vi "ConsoleRedErrors.vi"(8 "Text.Selection:End":u32, 9 "Front Panel":refnum<vi>, 10 "Console in":string, 11 "String in":refnum<vi>) -> (2 "Array":T1(array[cluster]), 3 "Console":string)   [LabVIEW 2021]
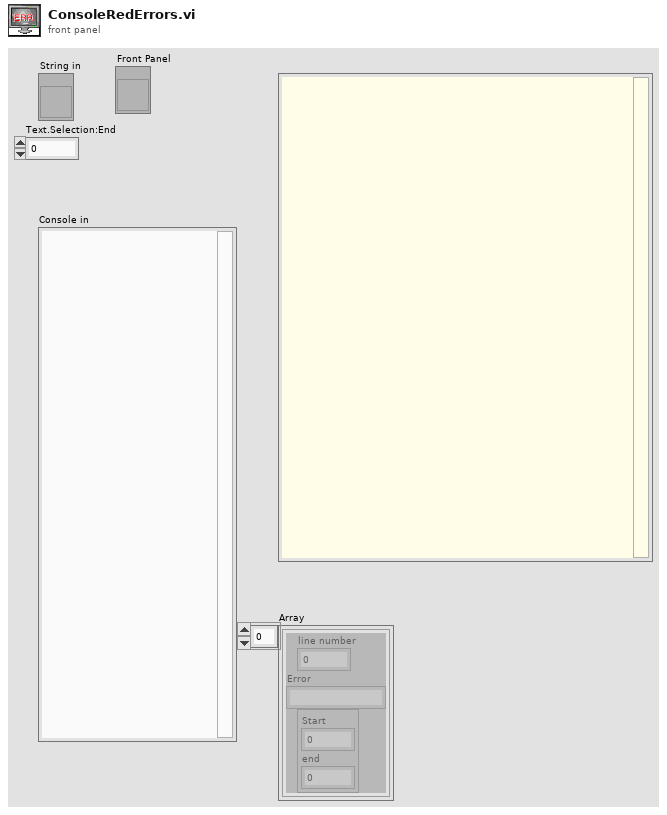
[diagram p1: front panel]
types:
  T1 = cluster{"line number":i32, "Error":string, cluster{"Start":i32, "end":i32}}[]
  T2 = cluster{i32, "Console in":string, cluster{i32, "offset past match":i32}}
  T3 = cluster{"line number":i32, "Error":string, cluster{"Start":i32, "end":i32}}
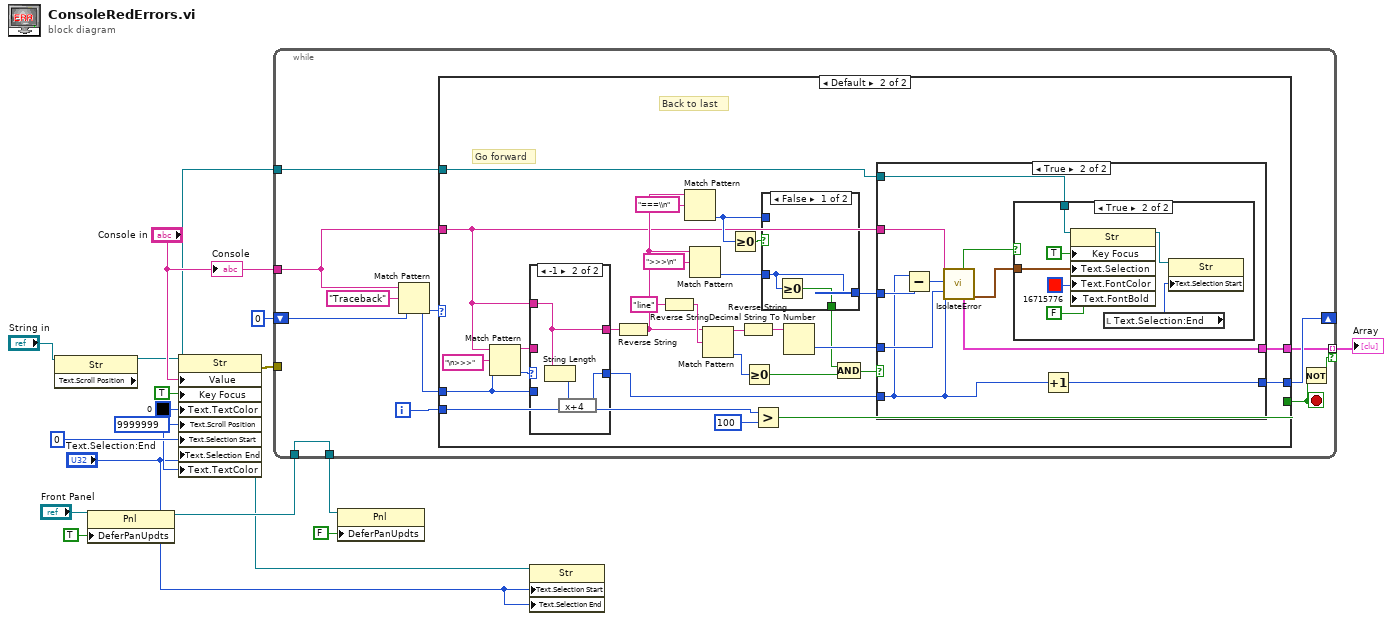
[diagram p0: block diagram]
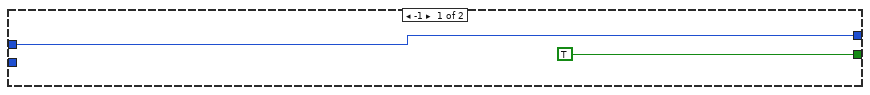
[diagram p2: hidden frame]
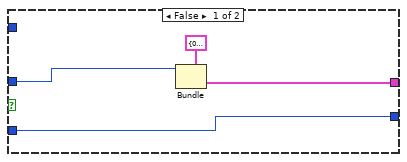
[diagram p3: hidden frame]
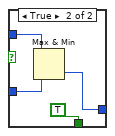
[diagram p6: hidden frame]
diagram:
  w3 = u32 0 ("Text.Text Colors:Text Color")
  n1 = property on="Property Node" class="Str" props=["Text", "Scroll Position"](reference="String in") -> (reference out=w10:refnum<vi>)  [unwired: 1 in, 2 out]
  n2 = property class="Pnl"(reference="Front Panel", "DeferPanUpdts"=TRUE ("Defer Panel Updates")) -> (reference out=w5:refnum<vi>)  [unwired: 1 in, 1 out]
  n3 = property on="Property Node" class="Str"(reference=w10, "Value"="Console in", "Key Focus"=TRUE, "Text.TextColor"=w3, "Text.Scroll Position"=u32 9999999, "Text.Selection Start"=u32 0 ("Text.Selection:Start"), "Text.Selection End"="Text.Selection:End", "Text.TextColor"=w3) -> (reference out=w2:refnum<vi>, error out=w14:errorcluster)  [unwired: 1 in]
  n4 = while {
    tunnel: "Console in" -> [w27]
    shift-right: [w25] -> _
    shift-left: 0 ("offset past match") -> [w26]
    tunnel: [w23] -> w16 mode=indexing if=w21
    tunnel: w14 -> [_]
    tunnel: w10 -> [w19]
    tunnel: [w18] -> w6
    tunnel: w5 -> [w18]
    i -> [w20]
    stop <- w22 stop-if-true
    n5 = Match Pattern(string=w27, regular expression="Traceback", offset (0)=w26) -> (offset past match=w24:i32)  [unwired: 3 out]
    n6 = case shown="Default" w24 {
      tunnel: w24 -> [w29 w32]
      tunnel: w27 -> [_ w35]
      tunnel: [w29 w46] -> w25
      tunnel: [TRUE w43] -> w22
      tunnel: [_ w52] -> w23
      tunnel: w20 -> [_ w44]
      tunnel: w19 -> [_ w31]
      frame -1 {
      }
      frame Default {
        # "Back to last"
        # "Go forward"
        n7 = Match Pattern(string=w35, regular expression="\n>>>", offset (0)=w32) -> (before substring=w33:string, offset past match=w37:i32)  [unwired: 2 out]
        n8 = case shown="-1" w37 {
          selector: w37 -> [w81 _]
          tunnel: [w82 w85] -> w36
          tunnel: w35 -> [_ w85]
          tunnel: [w81 w83] -> w34
          tunnel: w33 -> [w82 _]
          tunnel: w32 -> [_ _]
          frame Default {
          }
          frame -1 {
            n9 = String Length(string=w85) -> (length=w84:i32)
            n10 = expression code="x+4"(w84) -> (w83:i32)
          }
        }
        n11 = Reverse String(1:w36) -> (0:w50:string)
        n12 = Reverse String(1:"line" ("regular expression")) -> (0:w57:string)
        n13 = Match Pattern(string=w50, regular expression="===\\n") -> (offset past match=w49:i32)  [unwired: 1 in, 3 out]
        n14 = Match Pattern(string=w50, regular expression=">>>\n") -> (offset past match=w39:i32)  [unwired: 1 in, 3 out]
        n15 = Match Pattern(string=w50, regular expression=w57) -> (before substring=w56:string, offset past match=w42:i32)  [unwired: 1 in, 2 out]
        n16 = Greater Or Equal To 0?(x=w49) -> (x >= 0?=w48:bool)
        n17 = Reverse String(1:w56) -> (0:w55:string)
        n18 = Greater Or Equal To 0?(x=w42) -> (x >= 0?=w41:bool)
        n19 = Greater?(x=w44, y=100) -> (0:w43:bool)
        n20 = case shown="False" w48 {
          tunnel: w39 -> [w87 w91]
          tunnel: w49 -> [_ w90]
          tunnel: [w87 w89] -> w47
          tunnel: [w86 TRUE] -> w38
          frame False {
            n21 = Greater Or Equal To 0?(x=w87) -> (x >= 0?=w86:bool)
          }
          frame True {
            n22 = Max & Min(x=w90, y=w91) -> (min(x,y)=w89:i32)  [unwired: 1 out]
          }
        }
        n23 = Decimal String To Number(string=w55) -> (number=w53:i32)  [unwired: 2 in, 1 out]
        n24 = Compound Arithmetic op=AND(w38, w41) -> (w40:bool)
        n25 = case shown="True" w40 {
          tunnel: w35 -> [_ w73]
          tunnel: w53 -> [w62 w70]
          tunnel: [w60 w67] -> w52
          tunnel: w47 -> [_ w72]
          tunnel: [w63 w71] -> w46
          tunnel: w34 -> [w63 w64]
          tunnel: w31 -> [_ w65]
          frame False {
            n26 = Bundle(cluster=T2 {0, "Console in"="", {0, "offset past match"=0}}, w62) -> (w60:T2)  [unwired: 2 in]
          }
          frame True {
            n27 = Subtract(x=w64, y=w72) -> (x-y=w66:i32)
            n28 = call "IsolateError.vi"("Err Line"=w64, "Number of lines"=w70, "start"=w66, "Console in"=w73) -> ("line coord"=w68:cluster{"Start":i32, "end":i32}, "Line info"=w67:T3, "success?"=w69:bool)  [unwired: 2 in, 3 out]
            n29 = case shown="True" w69 {
              tunnel: w68 -> [_ w77]
              tunnel: w65 -> [_ w76]
              frame False {
              }
              frame True {
                n30 = property on="Property Node" class="Str"(reference=w76, "Key Focus"=TRUE, "Text.Selection"=w77, "Text.FontColor"=u32 16715776 ("Text.Text Colors:Text Color"), "Text.FontBold"=FALSE ("Text.Font:Bold")) -> (reference out=w75:refnum<vi>)  [unwired: 1 in, 1 out]
                n31 = local read "Text.Selection:End"() -> (w74:u32)
                n32 = property on="Property Node" class="Str"(reference=w75, "Text.Selection Start"=w74) -> ()  [unwired: 1 in, 2 out]
              }
            }
            n33 = Increment(x=w64) -> (x+1=w71:i32)
          }
        }
      }
    }
    n34 = Not(x=w22) -> (.not. x?=w21:bool)
  }
  "Array" <- w16
  n35 = property class="Pnl"(reference=w6, "DeferPanUpdts"=FALSE ("Defer Panel Updates")) -> ()  [unwired: 1 in, 2 out]
  n36 = property on="Property Node" class="Str"(reference=w2, "Text.Selection Start"="Text.Selection:End", "Text.Selection End"="Text.Selection:End") -> ()  [unwired: 1 in, 2 out]
  "Console" <- "Console in"
